vi "Cal-MotorStack Status.vi"(6 "StageSelection":enum16{"X-Y", "Z"}(ring), 9 "Timed out while waiting for acknowledgement in":bool, 10 "Last State":T1=enum."Motor Zstack-STOP", 11 "Initial motor position (um)":sgl) -> (1 "Motor timed out or errored out":bool, 2 "Cancelled":bool, 3 "Measured cal value":sgl)   [LabVIEW 2020]
uses:
  Typedefs/Top level VI states.ctl
  AOL Z/Typedefs/Cal mode.ctl
  Globals/gl_Calibration globals.vi
  Global Variables/General Globals.vi
panel:
  in  "Max offset (us)":i32=10 min=5 max=100
  in  "Wait before measurement (ms)":u32=500
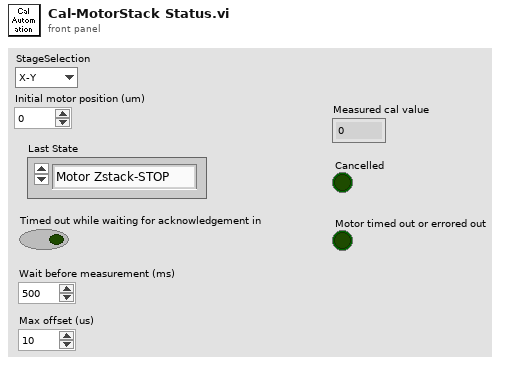
[diagram p1: front panel]
types:
  T1 = typedef "Top level VI states.ctl" = enum16{"None", "Initialise UI", "<STACK PROTOCOL STATES>", "AOL Zstack-START", "AOL Zstack-STOP", "Motor Zstack-START", "Motor Zstack-STOP", "<ACQUISITION PROTOCOL STATES> ", "Functional Acquisition-START", "Functional Acquisition-STOP", "Single Plane Acquisition-START", "Single Plane Acquisition-STOP", "Volume Acquisition-START", "Volume Acquisition-STOP", "<LIVE IMAGING PROTOCOL STATES>", "Live Imaging-START", "Live Imaging-STOP", "Live Plane Imaging-START", "Live Plane Imaging-STOP", "Live Volume Imaging-START", "Live Volume Imaging-STOP", "<MOVEMENT CORRECTION PROTOCOL STATES>", "EXIT"}
  T2 = typedef "Cal mode.ctl" = enum16{"Automatic", "Interactive"}
  T3 = typedef "AOL Z cal process refs.ctl" = cluster{"This VI":refnum<vi>, "Abort (ind)":refnum<vi>, "Next (ind)":refnum<vi>, "Cancel":refnum<vi>, "Next":refnum<vi>, "Message":refnum<vi>, "Progress":refnum<vi>}
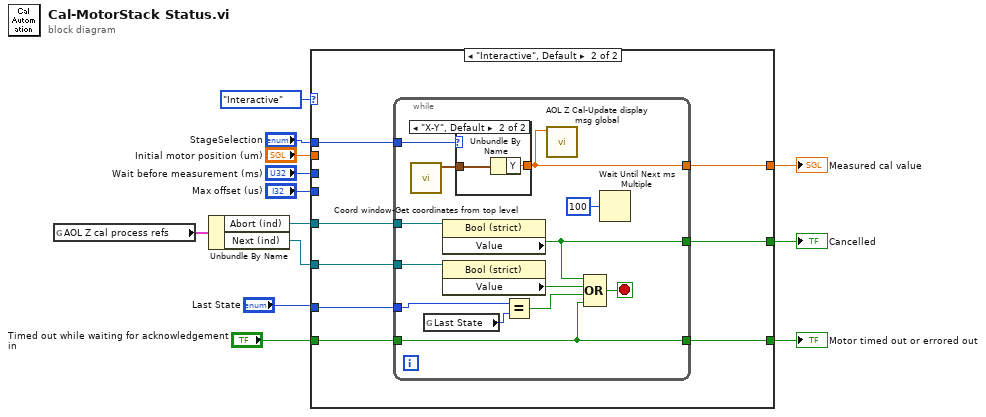
[diagram p0: block diagram]
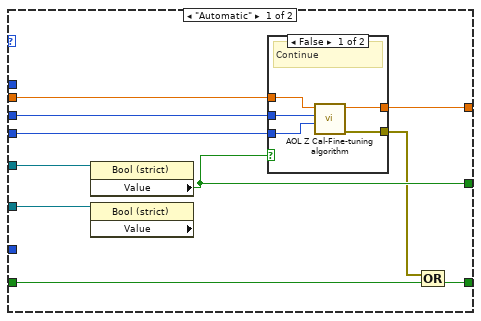
[diagram p2: hidden frame]
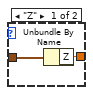
[diagram p4: hidden frame]
diagram:
  n1 = global read "gl_Calibration globals.vi" "AOL Z cal process refs"() -> (w7:T3)
  n2 = Unbundle By Name(w7) -> ("Abort (ind)"=w12:refnum<vi>, "Next (ind)"=w13:refnum<vi>)
  n3 = case shown="\"Interactive\", Default" Cal_mode."Interactive" ("Calibration Mode") {
    tunnel: w13 -> [w23 w36]
    tunnel: w12 -> [w22 w35]
    tunnel: "Initial motor position (um)" -> [w21 _]
    tunnel: [w20 w34] -> w10
    tunnel: "Timed out while waiting for acknowledgement in" -> [w19 w33]
    tunnel: [w18 w32] -> w8
    tunnel: "Wait before measurement (ms)" -> [w17 _]
    tunnel: [w16 w31] -> w5
    tunnel: "Max offset (us)" -> [w15 _]
    tunnel: "StageSelection" -> [_ w30]
    tunnel: "Last State" -> [_ w29]
    frame "Automatic" {
      n4 = property class="Bool (strict)"(reference=w22) -> ("Value"=w18:bool)  [unwired: 1 in, 2 out]
      n5 = property class="Bool (strict)" props=["Value"](reference=w23) -> ()  [unwired: 1 in, 3 out]
      n6 = case shown="False" w18 {
        tunnel: w21 -> [w28 _]
        tunnel: w17 -> [w27 _]
        tunnel: [w26 _] -> w16
        tunnel: [w25 _] -> w14
        tunnel: w15 -> [w24 _]
        frame False {
          # "Continue"
          n7 = call "AOL Z Cal-Fine-tuning algorithm.vi"("Max offset (us)"=w24, "Wait before measurement (ms)"=w27, "Initial motor position (um)"=w28) -> ("error out"=w25:errorcluster, "Measured cal value"=w26:sgl)  [unwired: 7 in]
        }
        frame True {
          # "Abort"
        }
      }
      n8 = Compound Arithmetic op=OR(w14, w19) -> (w20:bool)
    }
    frame "Interactive", Default {
      n9 = while {
        tunnel: w36 -> [w49]
        tunnel: w35 -> [w48]
        tunnel: [w40] -> w34
        tunnel: w33 -> [w40]
        tunnel: [w47] -> w32
        tunnel: [w42] -> w31
        tunnel: w30 -> [w41]
        tunnel: w29 -> [w37]
        stop <- w45 stop-if-true
        n10 = call "Coord window-Get coordinates from top level.vi"() -> ("Coordinates"=w43:cluster{"X":sgl, "Y":sgl, "Z":sgl})  [unwired: 11 in]
        n11 = global read "General Globals.vi" "Last State"() -> (w38:T1)
        n12 = property class="Bool (strict)"(reference=w48) -> ("Value"=w47:bool)  [unwired: 1 in, 2 out]
        n13 = property class="Bool (strict)"(reference=w49) -> ("Value"=w46:bool)  [unwired: 1 in, 2 out]
        n14 = case shown="\"X-Y\", Default" w41 {
          tunnel: w43 -> [w51 w53]
          tunnel: [w50 w52] -> w42
          frame "Z" {
            n15 = Unbundle By Name(w51) -> ("Z"=w50:sgl)
          }
          frame "X-Y", Default {
            n16 = Unbundle By Name(w53) -> ("Y"=w52:sgl)
          }
        }
        n17 = Equal?(x=w37, y=w38) -> (x = y?=w39:bool)
        n18 = call "AOL Z Cal-Update display msg global.vi"("Motor Z"=w42) -> ()  [unwired: 11 in]
        n19 = Compound Arithmetic op=OR(w47, w46, w39, w40) -> (w45:bool)
        n20 = Wait Until Next ms Multiple(millisecond multiple=u32 100) -> ()  [unwired: 1 out]
      }
    }
  }
  "Motor timed out or errored out" <- w10
  "Cancelled" <- w8
  "Measured cal value" <- w5
